vi "sub_Generate_Packet_Array.vi"(0 "user  bitstream":i8[](array[numeric]), 1 "PN sequence order\nfor Sync":i32=9 caption="PN sequence order (9)", 5 "Packet Parameters":T1, 7 "Packet Number":i32, 9 "Cyclic Padding Bits":i32) -> (4 "Output Packet":i8[](array[numeric]))   [LabVIEW 2015]
uses:
  <vilib>/addons/Modulation/Digital/General/MT Generate Bits (Galois, PN Order).vi
  <vilib>/addons/Modulation/Digital/Support/Common/Validators/mod_Generate Bits Validate.vi
  <vilib>/addons/Modulation/Analog/support/mod_Set Error Source.vi
  <vilib>/addons/Modulation/Digital/General/subVIs/mod_Generate Bits PN Sequence.vi
  <vilib>/addons/Modulation/niDMT.lvlib
panel:
  out "error out":errorcluster
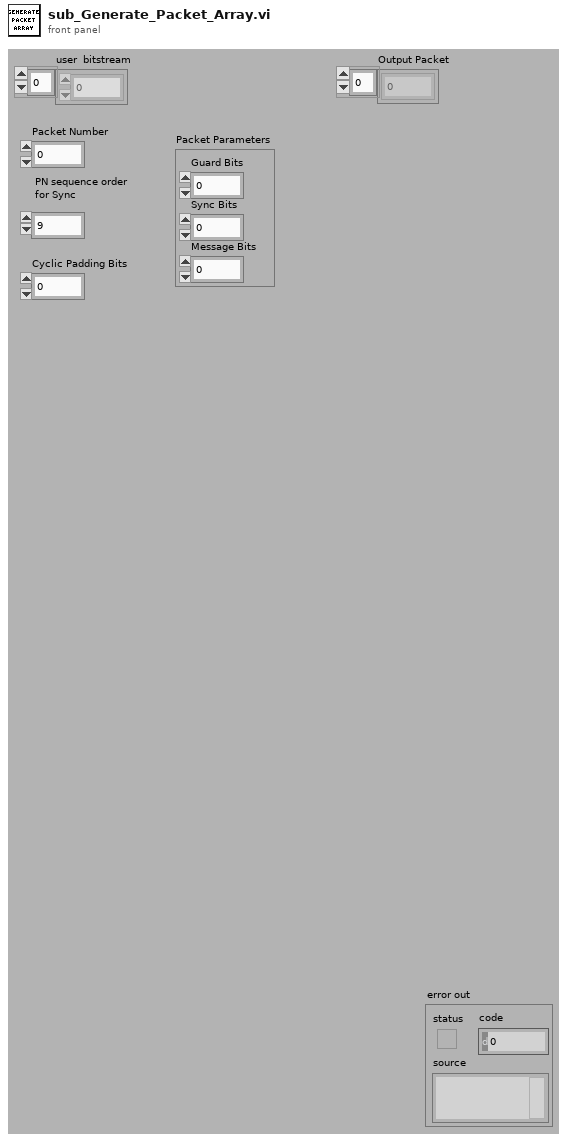
[diagram p1: front panel]
types:
  T1 = cluster{"Guard Bits ":i32, "Sync Bits":i32, "Message Bits":i32}
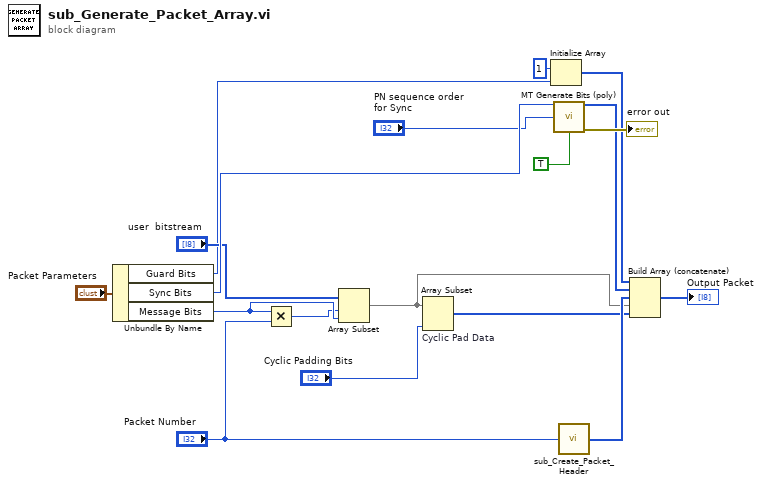
[diagram p0: block diagram]
diagram:
  n1 = Unbundle By Name("Packet Parameters") -> ("Guard Bits"=w5:i32, "Sync Bits"=w15:i32, "Message Bits"=w13:i32)
  n2 = Multiply(x=w13, y="Packet Number") -> (x*y=w2:i32)
  n3 = Array Subset(array="user  bitstream", index=w2, length=w13) -> (w1:i8[])
  n4 = Array Subset "Cyclic Pad Data"(array=w1, length="Cyclic Padding Bits") -> (w6:i8[])  [unwired: 1 in]
  n5 = Initialize Array(i8 1 ("Numeric"), w5) -> (w3:i8[])
  n6 = call-poly <vilib>:"MT Generate Bits (poly).vi"("total bits (128)"=w15, "PN sequence order (9)"="PN sequence order\nfor Sync", "reset? (T)"=TRUE ("Reset? (T)")) -> ("output bit stream"=w10:i8[], "error out"=→"error out":errorcluster)  [unwired: 10 in, 1 out]
  n7 = call "sub_Create_Packet_Header.vi"("Packet Number"="Packet Number") -> ("header bits"=w14:i8[])
  n8 = Build Array (concatenate)(w3, w10, w14, w1, w6) -> (→"Output Packet":i8[])
